vi "Get Name.vi"(8 "error in (no error)":errorcluster, 11 "Object in":refnum<class "Object.lvclass">) -> (0 "error out":errorcluster, 2 "Name":string, 3 "Object out":refnum<class "Object.lvclass">)   [LabVIEW 2019, in "HierDAL Library.lvlib" / "Models.lvlib" / "Object.lvclass"]
uses:
  Object.lvclass
  Object.lvclass/Object.ctl
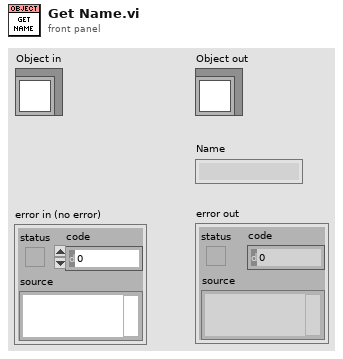
[diagram p1: front panel]
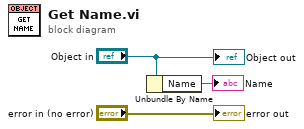
[diagram p0: block diagram]
diagram:
  n1 = Unbundle By Name("Object in") -> ("Name"=→"Name":string)
  "error out" <- "error in (no error)"
  "Object out" <- "Object in"
